vi "Wait Client Loops Running.vi"(8 "error in (no error)":errorcluster, 11 "TCPMessaging in":refnum<class "TCPMessaging.lvclass">) -> (0 "error out":errorcluster, 2 "Closing":bool, 3 "TCPMessaging out":refnum<class "TCPMessaging.lvclass">)   [LabVIEW 2020, in "Vecto.lvlib" / "TCPMessaging.lvclass"]
uses:
  TCPMessaging.lvclass
  TCPMessaging.lvclass/TCPMessaging.ctl
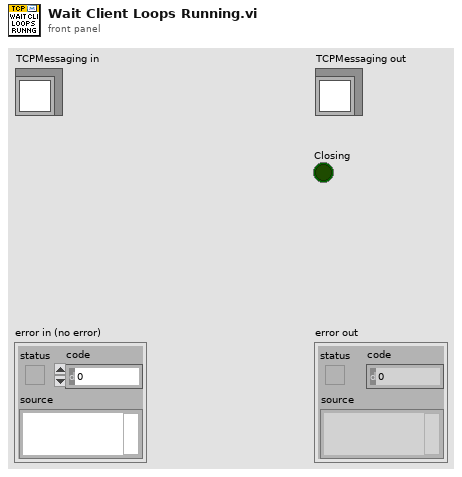
[diagram p1: front panel]
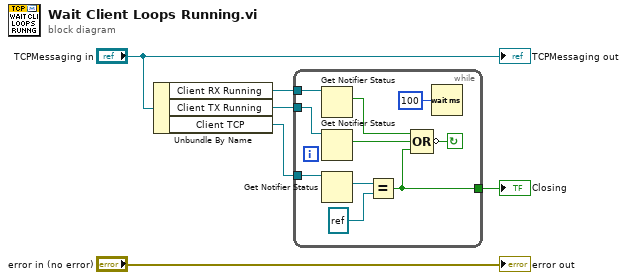
[diagram p0: block diagram]
diagram:
  n1 = Unbundle By Name("TCPMessaging in") -> ("Client RX Running"=w5:refnum<notifier>, "Client TX Running"=w4:refnum<notifier>, "Client TCP"=w2:refnum<notifier>)
  n2 = while {
    tunnel: w5 -> [w15]
    tunnel: w4 -> [w16]
    tunnel: w2 -> [w12]
    tunnel: [w9] -> w1
    stop <- w14 continue-if-true
    n3 = Get Notifier Status(notifier=w15) -> (current notification=w8:bool)  [unwired: 1 in, 4 out]
    n4 = Get Notifier Status(notifier=w16) -> (current notification=w7:bool)  [unwired: 1 in, 4 out]
    n5 = Get Notifier Status(notifier=w12) -> (current notification=w11:refnum<k5>)  [unwired: 1 in, 4 out]
    n6 = Equal?(x=w11, y=refnum<k5> refnum) -> (x = y?=w9:bool)
    n7 = Compound Arithmetic op=OR(w8, w7, w9) -> (invert w14:bool)
    n8 = Wait (ms)(milliseconds to wait=u32 100) -> ()  [unwired: 1 out]
  }
  "Closing" <- w1
  "error out" <- "error in (no error)"
  "TCPMessaging out" <- "TCPMessaging in"
